vi "LockinDAQ.TestLauncher.vi"() -> ()   [LabVIEW 2016, in "LockinDAQ.lvclass"]
uses:
  LockinDAQ.lvclass
  <vilib>/JKI/JKI SMO/SMO/SMO.lvclass
  <vilib>/JKI/JKI SMO/SMO/Typedefs/SMOState --Enum.ctl
  Typedefs/Set State-enum.ctl
  Instrument.Lockin/Instrument.Lockin.lvclass
  C:/Program Files (x86)/National Instruments/LabVIEW 2019/vi.lib/JKI/JKI SMO/SMO/SMO.lvclass
  Typedefs/Function-enum.ctl
  Typedefs/AO-cluster.ctl
  Typedefs/REF-cluster.ctl
  Typedefs/446xAO-enum.ctl
  Typedefs/AO.config(UI)-cluster.ctl
  Typedefs/AO.config(UI)-array.ctl
  Typedefs/AI.coupling-enum.ctl
  Typedefs/446xAI-enum.ctl
  Typedefs/AI.config(UI)-cluster.ctl
  Typedefs/AI.config(UI)-array.ctl
  Typedefs/Sampling.ctl
  Typedefs/Sample Mode--Ring.ctl
  Typedefs/State-enum.ctl
panel:
  out "DAQ state":T1=enum."created"
  in  "Tab Control 2":T2(tab)=enum."AI"
  out "AO":waveform(dbl)[](graph)
  out "AI":waveform(dbl)[](graph)
  out "WFM 3":waveform(dbl)[](graph)
  out "REF":waveform(dbl)[](graph)
  out "Results":dbl(graph)
  in  "Reset DAQ":bool
  in  "Stop DAQ":bool
  in  "Start DAQ":bool
  in  "Tab Control":enum32{"Output", "REF", "DAQ"}(tab)=enum."DAQ"
  in  "Channels: AO":T3={"Ch"=[], "Amp (V)"=[0.01, 0.0, 0.0, 0.0, 0.0, 0.0, 0.0, 0.0], "DC (V)"=[0.0, 0.0, 0.0, 0.0, 0.0, 0.0, 0.0, 0.0], "f (Hz)"=[0.0, 0.0, 0.0, 0.0, 0.0, 0.0, 0.0, 0.0], "Phase (°)"=[13.1, 13.0, 13.0, 13.0, 13.0, 13.0, 13.0, 13.0], "Function"=[enum."Sine", enum."Sine", enum."Sine", enum."Sine", enum."Sine", enum."Sine", enum."Sine", enum."Sine"], "Sweep?"=[FALSE, FALSE, FALSE, FALSE, FALSE, FALSE, FALSE, FALSE]} {"f (Hz)" min=0.001 max=10000.0; "DC (V)" format="%.3p"; "Amp (V)" format="%.3p"}
  in  "Channels: Lockin":T5={"Ch"=[13], " f (Hz)"=[13.0], "Phase (°)"=[0.0], "TC (s)"=[0.0], "order"=[0]} {"order" min=1; "TC (s)" min=0.0001 format="%#_3p"; "Phase (°)" format="%.3g"; "f (Hz)" format="%.3g"}
  in  "Gain":dbl[](array[numeric])=[1.0, 1.0]
  in  "AO Configuration":T6=[{"AO.Range"=enum."±0.1 V", "AO.channels"="PXI1Slot2/ao0:1"}]
  in  "AI Configuration":T9=[{"AI.Coupling"=10050, "AI.channels"="PXI1Slot2/ai0:1", "AI.Range"=enum."±0.316 V"}] {"AI.Coupling" items=["AC"=10045, "DC"=10050, "GND"=10066]}
  in  "sampling":T13={"Fs"=204789.0, "#s"=15753}
  in  "sample mode":T14=10123 items=["Finite Samples"=10178, "Continuous Samples"=10123]
  out "SMO State":T15=enum."Stopped"
  out "error out":errorcluster
  in  "Stop":bool
  # "Basic SMO Test Launcher"
  # "For instructions on how to use the JKI State Machine Objects, examples and video tutorials, visit:\nhttp://jki.net/state-machine-objects/\n\nJKI State Machine Objects™\nhttp://jki.net/state-machine-objects/\nCopyright (C) 2005-2015, JKI <info@jki.net>\nALL RIGHTS RESERVED"
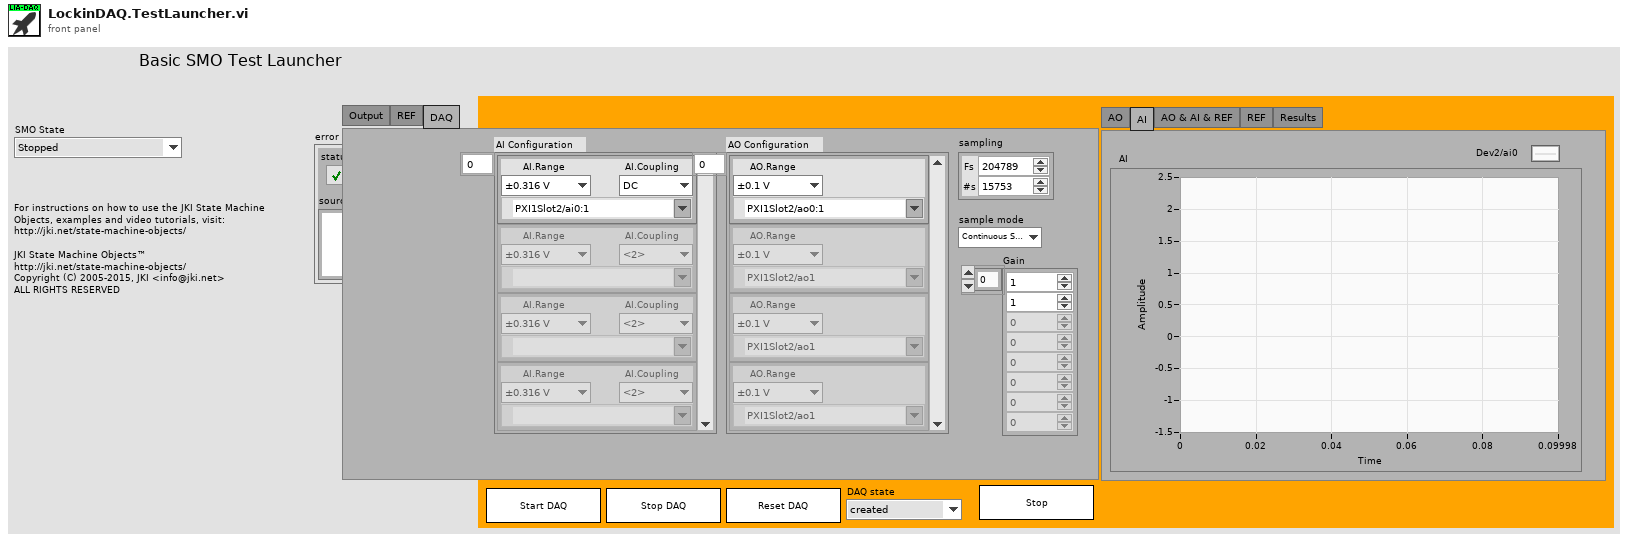
[diagram p1: front panel]
types:
  T1 = typedef "LockinDAQ.lvclass/State-enum.ctl" = enum16{"idle", "created", "started", "stopped", "sweeping"}
  T2 = enum32{"AO", "AI", "AO & AI & REF", "REF", "Results"}
  T3 = typedef "LockinDAQ.lvclass/AO-cluster.ctl" = cluster{"Ch":i32[], "Amp (V)":dbl[], "DC (V)":dbl[], "f (Hz)":dbl[], "Phase (°)":dbl[], "Function":T4[], "Sweep?":bool[]}
  T4 = typedef "LockinDAQ.lvclass/Function-enum.ctl" = enum16{"Sine", "Triangle", "Square", "Sawtooth"}
  T5 = typedef "LockinDAQ.lvclass/REF-cluster.ctl" = cluster{"Ch":i32[], " f (Hz)":dbl[], "Phase (°)":dbl[], "TC (s)":dbl[], "order":i32[]}
  T6 = typedef "LockinDAQ.lvclass/AO.config(UI)-array.ctl" = T7[]
  T7 = typedef "LockinDAQ.lvclass/AO.config(UI)-cluster.ctl" = cluster{"AO.Range":T8, "AO.channels":tag}
  T8 = typedef "LockinDAQ.lvclass/446xAO-enum.ctl" = enum16{"±0.1 V", "±1.0 V", "±10.0 V"}
  T9 = typedef "LockinDAQ.lvclass/AI.config(UI)-array.ctl" = T10[]
  T10 = typedef "LockinDAQ.lvclass/AI.config(UI)-cluster.ctl" = cluster{"AI.Coupling":T11, "AI.channels":tag, "AI.Range":T12}
  T11 = typedef "LockinDAQ.lvclass/AI.coupling-enum.ctl" = u16
  T12 = typedef "LockinDAQ.lvclass/446xAI-enum.ctl" = enum16{"±0.316 V", "±1.00 V", "±3.16 V", "±10.0 V", "±31.6 V", "±42.4 V"}
  T13 = typedef "LockinDAQ.lvclass/Sampling.ctl" = cluster{"Fs":dbl, "#s":i32}
  T14 = typedef "LockinDAQ.lvclass/Sample Mode--Ring.ctl" = i32
  T15 = typedef "SMO.lvclass/SMOState --Enum.ctl" = enum16{"unknown", "Created", "Started", "Stopped"}
  T16 = typedef "SMO.lvclass/Public Events.ctl" = cluster{"Error":refnum<user-event>, "State":refnum<user-event>, "Reserve State":refnum<user-event>}
  T17 = typedef "LockinDAQ.lvclass/PublicEvents--Cluster.ctl" = cluster{"getAO":refnum<user-event>, "getAI":refnum<user-event>, "getREF":refnum<user-event>, "getResults":refnum<user-event>, "getCalibration":refnum<user-event>, "getAOChannels":refnum<user-event>, "getREFChannels":refnum<user-event>, "getDAQState":refnum<user-event>, "getSweepResults":refnum<user-event>, "getIVSweepResults":refnum<user-event>}
  T18 = cluster{"Event Registration Refnum":refnum<event-registration>}
  T19 = typedef "LockinDAQ.lvclass/Set State-enum.ctl" = enum16{"start", "stop", "reset", "calibrate", "start sweep", "stop sweep"}
  T20 = typedef "LockinDAQ.lvclass/AI.config-array.ctl" = T21[]
  T21 = typedef "LockinDAQ.lvclass/AI.config-cluster.ctl" = cluster{"AI.channels":tag, "AI.Coupling":T11, "AI.Range":T12, "input terminal configuration":i32, "DAQ Type":T22}
  T22 = typedef "LockinDAQ.lvclass/DAQType-enum.ctl" = enum16{"None", "USB 4431", "PXI 446x"}
  T23 = typedef "LockinDAQ.lvclass/AO.config-array.ctl" = T24[]
  T24 = typedef "LockinDAQ.lvclass/AO.config-cluster.ctl" = cluster{"AO.channels":tag, "AO.Range":T8, "output terminal configuration":i32, "DAQ Type":T22}
  T25 = typedef "LockinDAQ.lvclass/PublicEvents--LockinDAQ.getAO.ctl" = waveform(dbl)[]
  T26 = typedef "LockinDAQ.lvclass/PublicEvents--LockinDAQ.getREF.ctl" = waveform(dbl)[]
  T27 = typedef "LockinDAQ.lvclass/PublicEvents--LockinDAQ.getAI.ctl" = waveform(dbl)[]
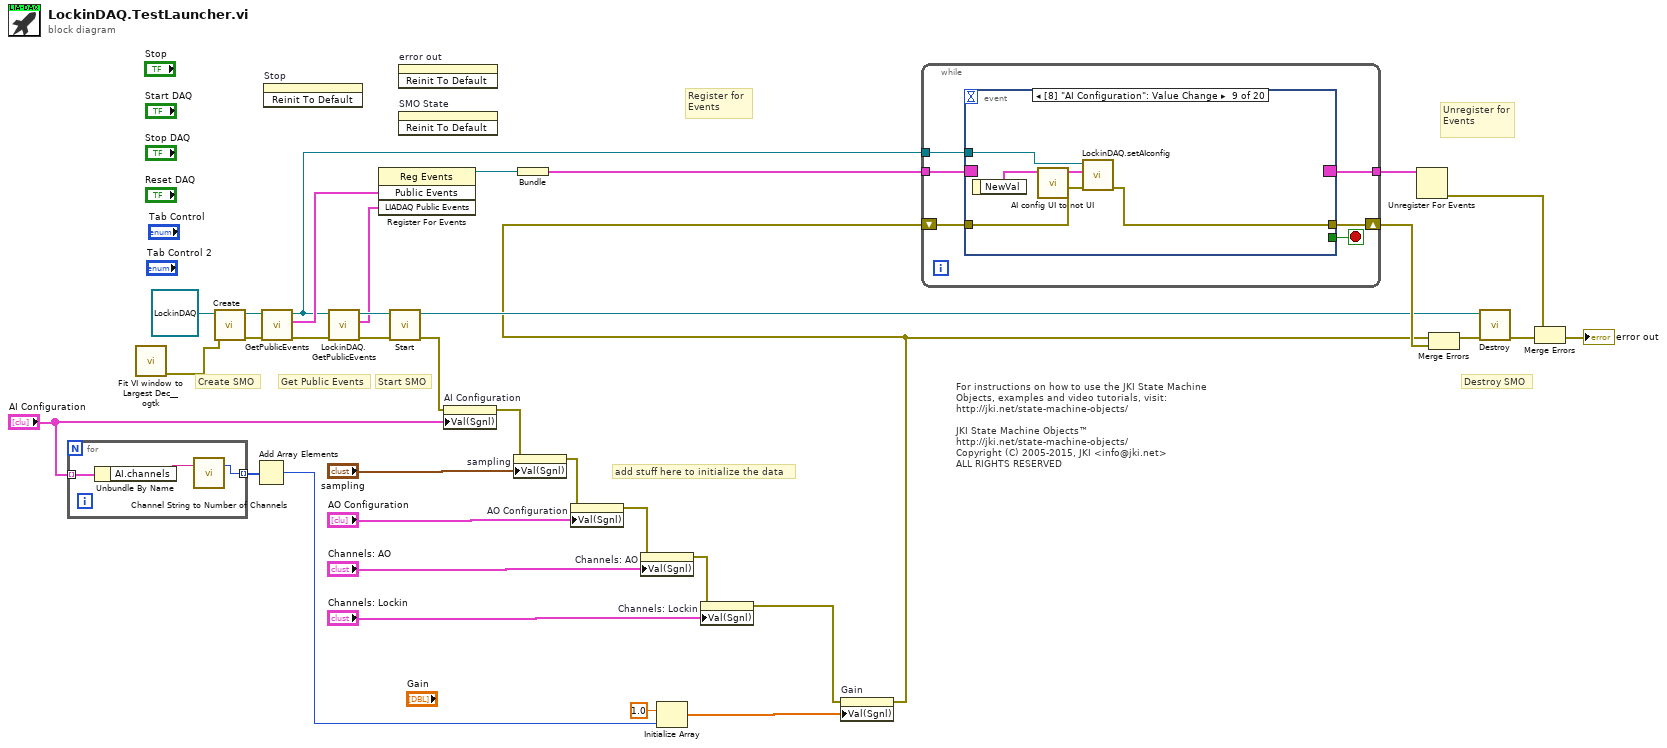
[diagram p0: block diagram]
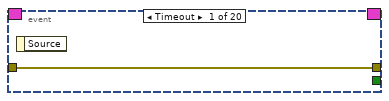
[diagram p2: hidden frame]
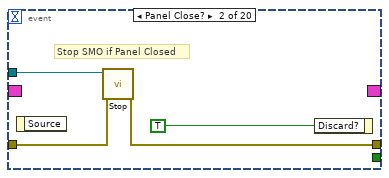
[diagram p3: hidden frame]
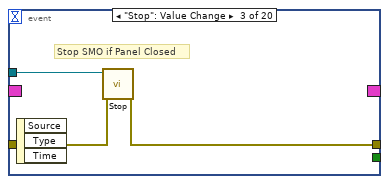
[diagram p4: hidden frame]
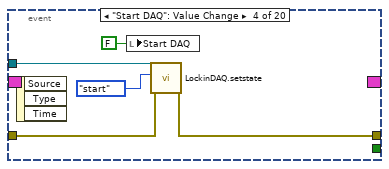
[diagram p5: hidden frame]
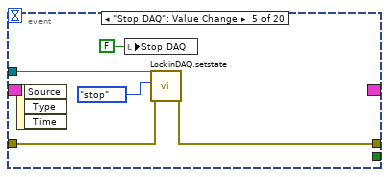
[diagram p6: hidden frame]
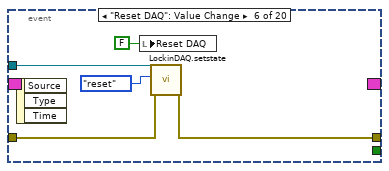
[diagram p7: hidden frame]
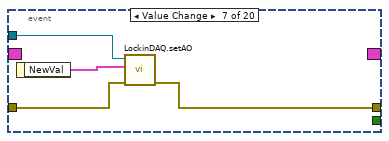
[diagram p8: hidden frame]
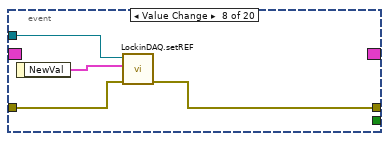
[diagram p9: hidden frame]
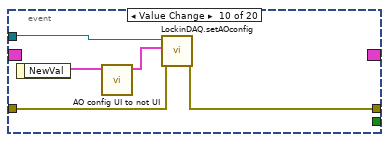
[diagram p10: hidden frame]
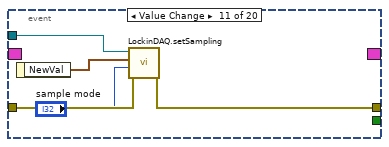
[diagram p11: hidden frame]
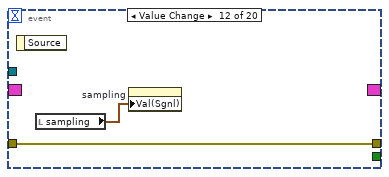
[diagram p12: hidden frame]
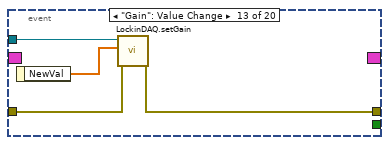
[diagram p13: hidden frame]
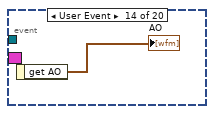
[diagram p14: hidden frame]
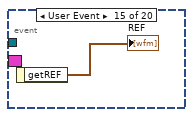
[diagram p15: hidden frame]
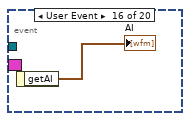
[diagram p16: hidden frame]
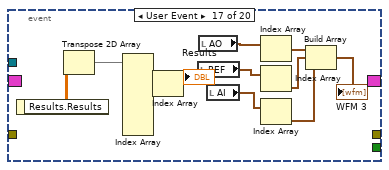
[diagram p17: hidden frame]
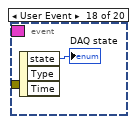
[diagram p18: hidden frame]
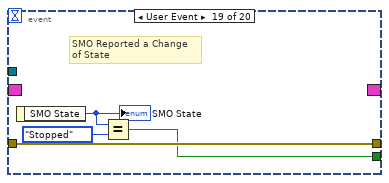
[diagram p19: hidden frame]
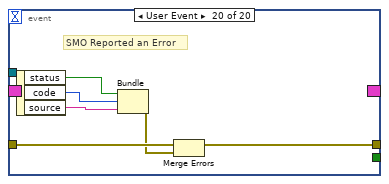
[diagram p20: hidden frame]
diagram:
  # "add stuff here to initialize the data"
  # "For instructions on how to use the JKI State Machine Objects, examples and video tutorials, visit:\nhttp://jki.net/state-machine-objects/\n\nJKI State Machine Objects™\nhttp://jki.net/state-machine-objects/\nCopyright (C) 2005-2015, JKI <info@jki.net>\nALL RIGHTS RESERVED"
  # "Get Public Events"
  # "Start SMO"
  # "Destroy SMO"
  # "Create SMO"
  # "Unregister for Events"
  # "Register for Events"
  n1 = for {
    tunnel: "AI Configuration" -> [w38] mode=indexing
    tunnel: [w36] -> w6 mode=indexing
    n2 = Unbundle By Name(w38) -> ("AI.channels"=w37:tag)
    n3 = call "Channel String to Number of Channels.vi"("Channels String"=w37) -> ("# channels"=w36:i32)  [unwired: 2 in]
  }
  n4 = call <userlib>:"Fit VI window to Largest Dec__ogtk.vi"() -> ("error out"=w18:errorcluster)  [unwired: 6 in, 1 out]
  n5 = call <vilib>:"Create.vi"("error in (no error)"=w18, "SMO"=refnum<class "LockinDAQ.lvclass"> refnum ("SMO.Template.lvclass")) -> ("error out"=w26:errorcluster, "SMO out"=w27:refnum<class "LockinDAQ.lvclass">)  [unwired: 7 in, 1 out]
  n6 = Add Array Elements(numeric array=w6) -> (sum=w3:i32)
  n7 = call <vilib>:"GetPublicEvents.vi"("error in (no error)"=w26, "SMO"=w27) -> ("error out"=w23:errorcluster, "Public Events"=w25:T16, "SMO out"=w22:refnum<class "LockinDAQ.lvclass">)  [unwired: 7 in]
  n8 = invoke on="Stop" class="Bool" method="Reinit To Default"() -> ()  [unwired: 3 in, 3 out]
  n9 = call "LockinDAQ.GetPublicEvents.vi"("error in (no error)"=w23, "LockinDAQ"=w22) -> ("error out"=w20:errorcluster, "LIADAQ Public Events"=w19:T17, "LockinDAQ out"=w21:refnum<class "LockinDAQ.lvclass">)  [unwired: 7 in]
  n10 = register-events(w25, w19) -> (reference out=w24:refnum<event-registration>)  [unwired: 2 in, 1 out]
  n11 = call <vilib>:"Start.vi"("error in (no error)"=w20, "SMO"=w21) -> ("error out"=w8:errorcluster, "SMO out"=w9:refnum<class "LockinDAQ.lvclass">)  [unwired: 8 in]
  n12 = invoke on="error out" class="Clust (strict)" method="Reinit To Default"() -> ()  [unwired: 3 in, 3 out]
  n13 = invoke on="SMO State" class="Enum (strict)" method="Reinit To Default"() -> ()  [unwired: 3 in, 3 out]
  n14 = property on="AI Configuration" class="Arr (strict)"(error in=w8, "Val(Sgnl)"="AI Configuration") -> (error out=w11:errorcluster)  [unwired: 1 in, 1 out]
  n15 = property on="sampling" class="Clust (strict)"(error in=w11, "Val(Sgnl)"="sampling") -> (error out=w12:errorcluster)  [unwired: 1 in, 1 out]
  n16 = Bundle("Event Registration Refnum"=w24) -> (w34:T18)  [unwired: 1 in]
  n17 = property on="AO Configuration" class="Arr (strict)"(error in=w12, "Val(Sgnl)"="AO Configuration") -> (error out=w13:errorcluster)  [unwired: 1 in, 1 out]
  n18 = property on="Channels: AO" class="Clust (strict)"(error in=w13, "Val(Sgnl)"="Channels: AO") -> (error out=w10:errorcluster)  [unwired: 1 in, 1 out]
  n19 = Initialize Array(1.0 ("element"), w3) -> (w4:dbl[])
  n20 = property on="Channels: Lockin" class="Clust (strict)"(error in=w10, "Val(Sgnl)"="Channels: Lockin") -> (error out=w1:errorcluster)  [unwired: 1 in, 1 out]
  n21 = property on="Gain" class="Arr (strict)"(error in=w1, "Val(Sgnl)"=w4) -> (error out=w2:errorcluster)  [unwired: 1 in, 1 out]
  n22 = while {
    shift-right: [w43] -> w33
    shift-left: w2 -> [w42]
    tunnel: w34 -> [w41]
    tunnel: [w40] -> w35
    tunnel: w22 -> [w39]
    stop <- w44 stop-if-true
    n23 = event shown="[8] \"AI Configuration\": Value Change" {
      selector: w41 -> [_ _ _ _ _ _ _ _ _ _ _ _ _ _ _ _ _ _ _ _]
      dyn-events: [_ _ _ _ _ _ _ _ _ _ _ _ _ _ _ _ _ _ _ _] -> w40
      timeout: _ -> [_ _ _ _ _ _ _ _ _ _ _ _ _ _ _ _ _ _ _ _]
      tunnel: [_ _ _ _ _ _ _ _ _ _ _ _ _ _ _ _ _ _ w112 _] -> w44
      tunnel: w39 -> [_ w49 w52 w57 w62 w67 w70 w74 w80 w81 w90 _ w96 _ _ _ _ _ _ _]
      tunnel: [w45 w48 w51 w56 w61 w66 w68 w72 w78 w82 w88 w91 w94 _ _ _ _ _ w115 w119] -> w43
      tunnel: w42 -> [w45 w47 w50 w55 w60 w65 w69 w73 w79 w83 w89 w91 w95 _ _ _ _ _ w115 w117]
      event Timeout {
        n24 = event-data() -> ()  [unwired: 1 in, 1 out]
      }
      event Panel Close? {
        # "Stop SMO if Panel Closed"
        n25 = event-data() -> ()  [unwired: 1 in, 1 out]
        n26 = call <vilib>:"Stop.vi"("error in (no error)"=w47, "SMO"=w49) -> ("error out"=w48:errorcluster)  [unwired: 8 in, 1 out]
        n27 = event-data("Discard?"=TRUE ("OK")) -> ()  [unwired: 1 in, 1 out]
      }
      event "Stop": Value Change {
        # "Stop SMO if Panel Closed"
        n28 = event-data() -> ()  [unwired: 1 in, 3 out]
        n29 = call <vilib>:"Stop.vi"("error in (no error)"=w50, "SMO"=w52) -> ("error out"=w51:errorcluster)  [unwired: 8 in, 1 out]
      }
      event "Start DAQ": Value Change {
        n30 = event-data() -> ()  [unwired: 1 in, 3 out]
        n31 = local write "Start DAQ"(FALSE ("Start DAQ")) -> ()
        n32 = call "LockinDAQ.setstate.vi"("error in (no error)"=w55, "State"=Set_State-enum."start" ("setState"), "LockinDAQ"=w57) -> ("error out"=w56:errorcluster)  [unwired: 7 in, 1 out]
      }
      event "Stop DAQ": Value Change {
        n33 = event-data() -> ()  [unwired: 1 in, 3 out]
        n34 = local write "Stop DAQ"(FALSE ("Stop DAQ")) -> ()
        n35 = call "LockinDAQ.setstate.vi"("error in (no error)"=w60, "State"=Set_State-enum."stop" ("setState"), "LockinDAQ"=w62) -> ("error out"=w61:errorcluster)  [unwired: 7 in, 1 out]
      }
      event "Reset DAQ": Value Change {
        n36 = event-data() -> ()  [unwired: 1 in, 3 out]
        n37 = local write "Reset DAQ"(FALSE ("Reset DAQ")) -> ()
        n38 = call "LockinDAQ.setstate.vi"("error in (no error)"=w65, "State"=Set_State-enum."reset" ("setState"), "LockinDAQ"=w67) -> ("error out"=w66:errorcluster)  [unwired: 7 in, 1 out]
      }
      event Value Change {
        n39 = event-data() -> ("NewVal"=w71:T3)  [unwired: 1 in]
        n40 = call "LockinDAQ.setAO.vi"("error in (no error)"=w69, "Channels: AO"=w71, "LockinDAQ"=w70) -> ("error out"=w68:errorcluster)  [unwired: 7 in, 1 out]
      }
      event Value Change {
        n41 = event-data() -> ("NewVal"=w75:T5)  [unwired: 1 in]
        n42 = call "LockinDAQ.setREF.vi"("error in (no error)"=w73, "Channels: Lockin"=w75, "LockinDAQ"=w74) -> ("error out"=w72:errorcluster)  [unwired: 7 in, 1 out]
      }
      event Value Change {
        n43 = event-data() -> ("NewVal"=w77:T9)  [unwired: 1 in]
        n44 = call "AI config UI to not UI.vi"("AI Config (UI)"=w77) -> ("AI Config"=w76:T20)  [unwired: 10 in]
        n45 = call "LockinDAQ.setAIconfig.vi"("error in (no error)"=w79, "AI Configuration"=w76, "LockinDAQ"=w80) -> ("error out"=w78:errorcluster)  [unwired: 7 in, 1 out]
      }
      event Value Change {
        n46 = event-data() -> ("NewVal"=w85:T6)  [unwired: 1 in]
        n47 = call "AO config UI to not UI.vi"("AO Config (UI)"=w85) -> ("AO Config"=w84:T23)  [unwired: 10 in]
        n48 = call "LockinDAQ.setAOconfig.vi"("error in (no error)"=w83, "AO Configuration"=w84, "LockinDAQ"=w81) -> ("error out"=w82:errorcluster)  [unwired: 7 in, 1 out]
      }
      event Value Change {
        n49 = event-data() -> ("NewVal"=w87:T13)  [unwired: 1 in]
        n50 = call "LockinDAQ.setSampling.vi"("error in (no error)"=w89, "Sample Mode"="sample mode", "Sampling"=w87, "LockinDAQ"=w90) -> ("error out"=w88:errorcluster)  [unwired: 6 in, 1 out]
      }
      event Value Change {
        n51 = event-data() -> ()  [unwired: 1 in, 1 out]
        n52 = local read "sampling"() -> (w92:T13)
        n53 = property on="sampling" class="Clust (strict)"("Val(Sgnl)"=w92) -> ()  [unwired: 2 in, 2 out]
      }
      event "Gain": Value Change {
        n54 = event-data() -> ("NewVal"=w93:dbl[])  [unwired: 1 in]
        n55 = call "LockinDAQ.setGain.vi"("error in (no error)"=w95, "setGain"=w93, "LockinDAQ"=w96) -> ("error out"=w94:errorcluster)  [unwired: 7 in, 1 out]
      }
      event User Event {
        n56 = event-data() -> ("get AO"=→"AO":T25)  [unwired: 1 in]
      }
      event User Event {
        n57 = event-data() -> ("getREF"=→"REF":T26)  [unwired: 1 in]
      }
      event User Event {
        n58 = event-data() -> ("getAI"=→"AI":T27)  [unwired: 1 in]
      }
      event User Event {
        n59 = event-data() -> ("Results.Results"=w109:dbl[][])  [unwired: 1 in]
        n60 = Transpose 2D Array(2D array=w109) -> (transposed array=w110:dbl[][])
        n61 = Index Array(array=w110) -> (element #1=w108:dbl[])  [unwired: 8 in, 3 out]
        n62 = Index Array(array=w108) -> (element=→"Results":dbl)  [unwired: 1 in]
        n63 = local read "REF"() -> (w105:waveform(dbl)[])
        n64 = local read "AO"() -> (w106:waveform(dbl)[])
        n65 = local read "AI"() -> (w104:waveform(dbl)[])
        n66 = Index Array(array=w106) -> (element=w103:waveform(dbl))  [unwired: 1 in]
        n67 = Index Array(array=w105) -> (element=w102:waveform(dbl))  [unwired: 1 in]
        n68 = Index Array(array=w104) -> (element=w100:waveform(dbl))  [unwired: 1 in]
        n69 = Build Array(w103, w102, w100) -> (→"WFM 3":waveform(dbl)[])
      }
      event User Event {
        n70 = event-data() -> ("state"=→"DAQ state":T1)  [unwired: 1 in, 2 out]
      }
      event User Event {
        # "SMO Reported a Change\nof State"
        n71 = event-data() -> ("SMO State"=w114:T15)  [unwired: 1 in]
        "SMO State" <- w114
        n72 = Equal?(x=w114, y=SMOState_--Enum."Stopped") -> (x = y?=w112:bool)
      }
      event User Event {
        # "SMO Reported an Error"
        n73 = event-data() -> ("status"=w118:bool, "code"=w121:i32, "source"=w120:string)  [unwired: 1 in]
        n74 = Bundle("status"=w118, "code"=w121, "source"=w120) -> (w116:errorcluster)  [unwired: 1 in]
        n75 = Merge Errors(w117, w116) -> (w119:errorcluster)
      }
    }
  }
  n76 = Unregister For Events(event registration refnum=w35) -> (error out=w32:errorcluster)  [unwired: 1 in]
  n77 = Merge Errors(w2, w33) -> (w28:errorcluster)
  n78 = call <vilib>:"Destroy.vi"("error in (no error)"=w28, "SMO"=w9) -> ("error out"=w30:errorcluster)  [unwired: 9 in]
  n79 = Merge Errors(w32, w30) -> (→"error out":errorcluster)
